vi "T_At_WireGen.vi"   [LabVIEW 2019]
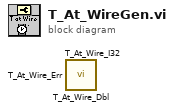
[diagram p0: block diagram]
diagram:
  n1 = call <userlib>:"T_At_Wire_Dbl.vi"() -> ()  [unwired: 10 in, 2 out]
  n2 = call <userlib>:"T_At_Wire_I32.vi"() -> ()  [unwired: 10 in, 2 out]
  n3 = call <userlib>:"T_At_Wire_Err.vi"() -> ()  [unwired: 10 in, 2 out]
